vi "Is Data Ready.vi"(8 "error in (no error)":errorcluster, 10 "Requested samples":i32, 11 "Red Pitaya Digitizer in":refnum<class "Red Pitaya Digitizer.lvclass">) -> (0 "error out":errorcluster, 1 "Data ready":bool, 2 "Availiable Samples":u32, 3 "Red Pitaya Digitizer out":refnum<class "Red Pitaya Digitizer.lvclass">)   [LabVIEW 2015]
uses:
  Red Pitaya Digitizer.lvclass
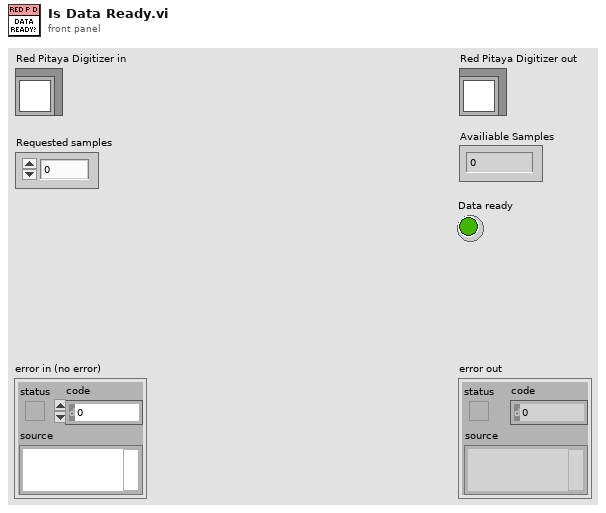
[diagram p1: front panel]
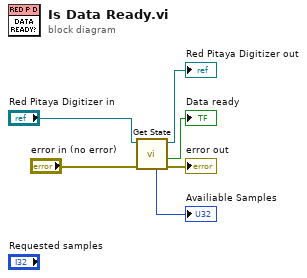
[diagram p0: block diagram]
diagram:
  n1 = call-dynamic "Get State.vi"("error in (no error)"="error in (no error)", "Red Pitaya Digitizer in"="Red Pitaya Digitizer in") -> ("error out"=→"error out":errorcluster, "Data ready"=→"Data ready":bool, "Red Pitaya Digitizer out"=→"Red Pitaya Digitizer out":refnum<class "Red Pitaya Digitizer.lvclass">, "Availiable Samples"=→"Availiable Samples":u32)  [unwired: 4 in, 2 out]
